vi "Main.vi"   [LabVIEW 2011]
uses:
  Classes/Actors/Controller/Controller.lvclass
  <userlib>/_Frameworks/ActorFramework/Message Queue/Message Queue.lvclass/Message Queue.ctl
  <userlib>/_Frameworks/ActorFramework/Message Queue/Message Queue.lvclass
  <userlib>/_Frameworks/ActorFramework/Actor/Actor.lvclass
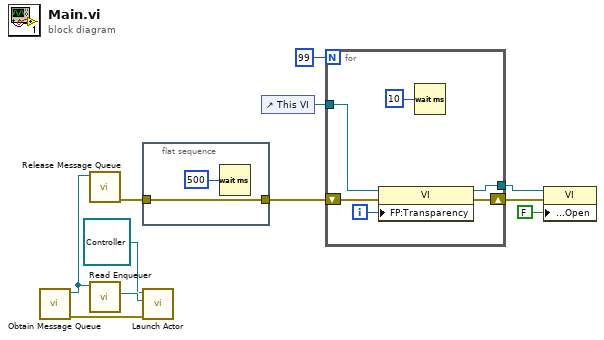
[diagram p0: block diagram]
diagram:
  n1 = call <userlib>:"Obtain Message Queue.vi"() -> ("error out"=w10:errorcluster, "Message Queue"=w9:refnum<class "Message Queue.lvclass">)  [unwired: 10 in]
  n2 = call <userlib>:"Release Message Queue.vi"("Message Queue"=w9) -> ("error out"=w1:errorcluster)  [unwired: 9 in, 1 out]
  n3 = call <userlib>:"Read Enqueuer.vi"("Message Queue"=w9) -> ("Message Enqueuer"=w11:refnum<class "Message Enqueuer.lvclass">)  [unwired: 10 in]
  n4 = flat-sequence {
    tunnel: [w13] -> w5
    tunnel: w1 -> [w13]
    frame #0 {
      n5 = Wait (ms)(milliseconds to wait=u32 500) -> ()  [unwired: 1 out]
    }
  }
  n6 = call <userlib>:"Launch Actor.vi"("error in (no error)"=w10, "Actor-to-Caller Enqueuer"=w11, "Actor"=refnum<class "Controller.lvclass"> refnum ("Controller.lvclass")) -> ()  [unwired: 7 in, 2 out]
  n7 = control-ref of="This VI"() -> (w7:refnum<vi>)
  n8 = for {
    N: 99 -> [_]
    tunnel: w7 -> [w19]
    tunnel: [w18] -> w6
    shift-right: [w16] -> w4
    shift-left: w5 -> [w17]
    i -> [w15]
    n9 = property class="VI"(reference=w19, error in=w17, "FP:Transparency"=w15) -> (reference out=w18:refnum<vi>, error out=w16:errorcluster)
    n10 = Wait (ms)(milliseconds to wait=u32 10) -> ()  [unwired: 1 out]
  }
  n11 = property class="VI"(reference=w6, error in=w4, "Front Panel.Open"=FALSE ("Front Panel Window:Open")) -> ()  [unwired: 2 out]
